vi "ActiveObjects_DynamicEvents.vi"(7 "Action":T2=enum."GeneratePattern", 8 "error in (no error)":errorcluster, 10 "DataIn":variant, 11 "ClassRefToActOn":refnum<vi>) -> (0 "error out":errorcluster, 1 "Name":string, 2 "DataOut":variant, 3 "Cancelled":bool)   [LabVIEW 2012]
uses:
  <resource>/Framework/Providers/Open_GDS/ClassProviders/Provider_BaseClassInterface/BaseProvider_SubVIs/BaseProvider_DesignPatternsActions.ctl
  <resource>/Framework/Providers/Open_GDS/ClassProviders/Common/LvClass_class/GDSLvClass_ProviderTypes.ctl
  <vilib>/picture/picture.llb/imagedata.ctl
  <resource>/Framework/Providers/Open_GDS/ClassProviders/Common/LvIcon_class/subvis/GDSLvIcon_TextDataType.ctl
  <resource>/Framework/Providers/Open_GDS/ClassProviders/Common/LvIcon_class/GDSLvIcon_WordCompressionType.ctl
  <resource>/Framework/Providers/Open_GDS/ClassProviders/Common/LvIcon_class/GDSLvIcon_TextAlignment.ctl
  <vilib>/Utility/lvfile.llb/NI_FileType.lvlib
panel:
  out "NameExist4":string
  in  "AddWindowControlVI":bool
  in  "WindowControlName":string caption="Enter process window control VI name"
  in  "ProcessCreation":T1(ring) caption="Process creation"
  out "NameExist1":string
  out "NameExist3":string
  out "NameExist2":string
  in  "AddInDestructor":bool
  in  "AddInConstructor":bool
  in  "StopName":string caption="Enter Stop Process Name"
  in  "StartName":string caption="Enter Start Process Name"
  in  "_Cancel":bool
  in  "_OK":bool
  in  "ProcessName":string caption="Enter Active Process Name"
  # "Active Object using Dymanic Events"
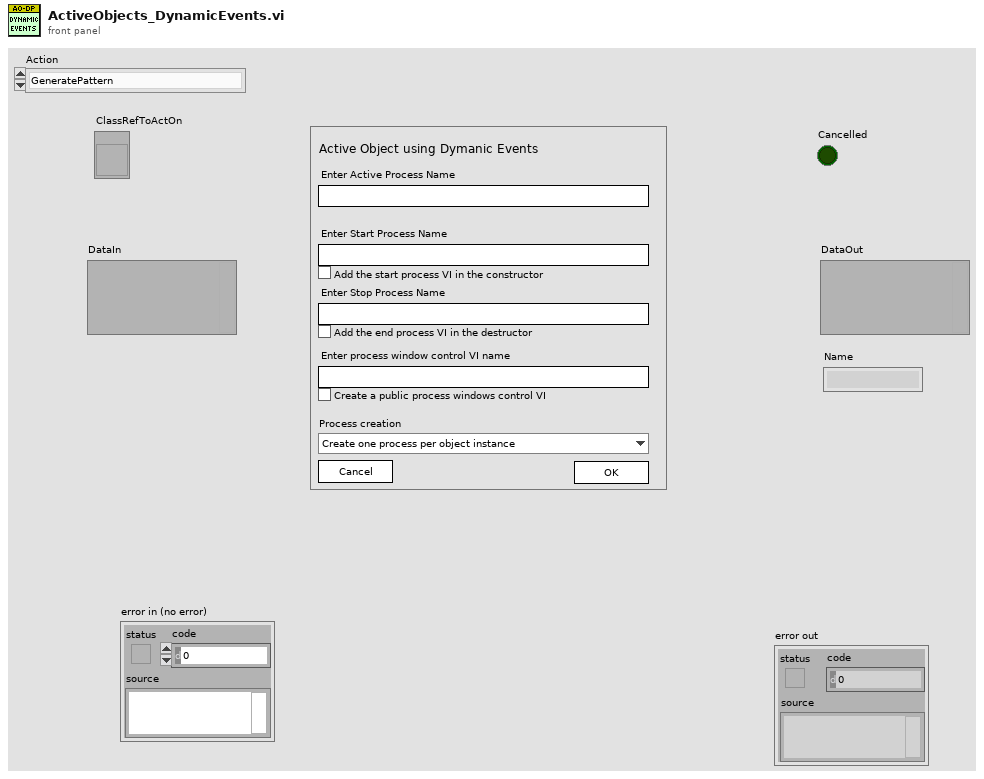
[diagram p1: front panel]
types:
  T1 = enum16{"Create one process per object instance", "Create only one process for this class"}
  T2 = typedef "BaseProvider_DesignPatternsActions.ctl" = enum16{"AddPatternDialog", "GeneratePattern", "RemovePattern", "CreatePatternMethod", "UpdatePattern"}
  T3 = typedef "GDSLvClass_ProviderTypes.ctl" = enum16{"UnKnown(LabVOOP)", "Native", "EndevoGOOP3", "OpenG(RootObject)", "OpenG(OpenG_Object)", "EndevoGOOP4", "JKI1"}
  T4 = cluster{"Data":cluster{"ProcessName":string, "StartName":string, "StopName":string, "AddInConstructor":bool, "AddInDestructor":bool, "ProcessCreation":enum16{"Create one process per object instance", "Create only one process for this class"}, "WindowControlName":string, "AddWindowControlVI":bool}, "ClassFolder":path, "SupportFolder":path, "ProcessCtl":refnum<vi>, "ProtectedFolder":refnum<vi>, "ProcessVI":refnum<vi>, "StartVI":refnum<vi>, "StopVI":refnum<vi>, "Application":refnum<vi>, "RepositoryVI":refnum<vi>, "ProcessIdRef":refnum<vi>, "ProcessRepository":path, "ClassProvider":T3, "TemplateName":string, "VI_ToFind":path, "MethodTemplate":path, "VI":refnum<vi>, "VI_ToFindSingleton":path, "Name":string, "WindowControlVI":refnum<vi>, "ClassType":enum16{"4x4x4", "6x8x6", "4x4x4_Singleton", "6x8x6_Singleton"}}
  T5 = cluster{"ProcessName":string, "StartName":string, "StopName":string, "AddInConstructor":bool, "AddInDestructor":bool, "ProcessCreation":enum16{"Create one process per object instance", "Create only one process for this class"}, "WindowControlName":string, "AddWindowControlVI":bool}
  T6 = cluster{"Cancelled":bool, "Files":path[], "ClassPath":path, "DataOut":variant, "Name":string}
  T7 = enum8{"Enabled", "Disabled", "Disabled and Grayed Out"}
  T8 = enum16{"4x4x4", "6x8x6", "4x4x4_Singleton", "6x8x6_Singleton"}
  T9 = enum32{"invalid VI type", "Standard VI", "Control VI", "Global VI", "Polymorphic VI", "Configuration VI", "SubSystem", "Facade VI", "Method VI"}
  T10 = typedef "GDSLvIcon_TextDataType.ctl" = cluster{"Text":string, "Allow Only Capital Chars":bool, "Compression":T11, "Alignment":T12}
  T11 = typedef "GDSLvIcon_WordCompressionType.ctl" = enum16{"Auto", "On", "Off"}
  T12 = typedef "GDSLvIcon_TextAlignment.ctl" = enum16{"Center", "Left", "Right"}
  T13 = typedef "imagedata.ctl" = cluster{"image type":i32, "image depth":i32, "image":u8[], "mask":u8[], "colors":u32[], "Rectangle":cluster{"left":i16, "top":i16, "right":i16, "bottom":i16}}
  T14 = typedef "GDSLvCLass_ClassSettingsType.ctl" = cluster{"ClassProviderName":string, "ClassTemplateUsed":string, "ClassTemplateVersion":string, "ClassDescription":string, "PlugIns":T15[], "ConnectorPanePattern":string}
  T15 = typedef "GDSLvClass_PlugIn.ctl" = cluster{"Type":T16, "ID":string, "Version":string, "Path":path, "Name":string, "Data":variant}
  T16 = typedef "GDSLvClass_PlugInTypes.ctl" = enum16{"DesignPattern", "MethodTypes"}
  T17 = enum32{"invalid scope", "public", "private", "protected"}[]
  T18 = enum16{"UINT8", "INT8", "UINT16", "INT16", "UINT32", "INT32", "UINT64", "INT64", "SGL", "DBL", "EXT", "CSG", "CDB", "CXT", "TimeStamp", "STRING", "PATH", "BOOL", "ENUM", "RefNum", "VIRefNum", "ClassRefNum", "Cluster", "Variant", "TypeRef", "Waveform", "LabVIEW Object", "Other"}[]
  T19 = typedef "GDSLvClass_IconSettingsType.ctl" = cluster{"Frame":u32, "Frame thickness":u8, "Header Background":u32, "Header Text":u32, "ColorPublic":u32, "ColorProtected":u32, "ColorPrivate":u32, "Body Text":u32, "ClassBodyIcon":string}
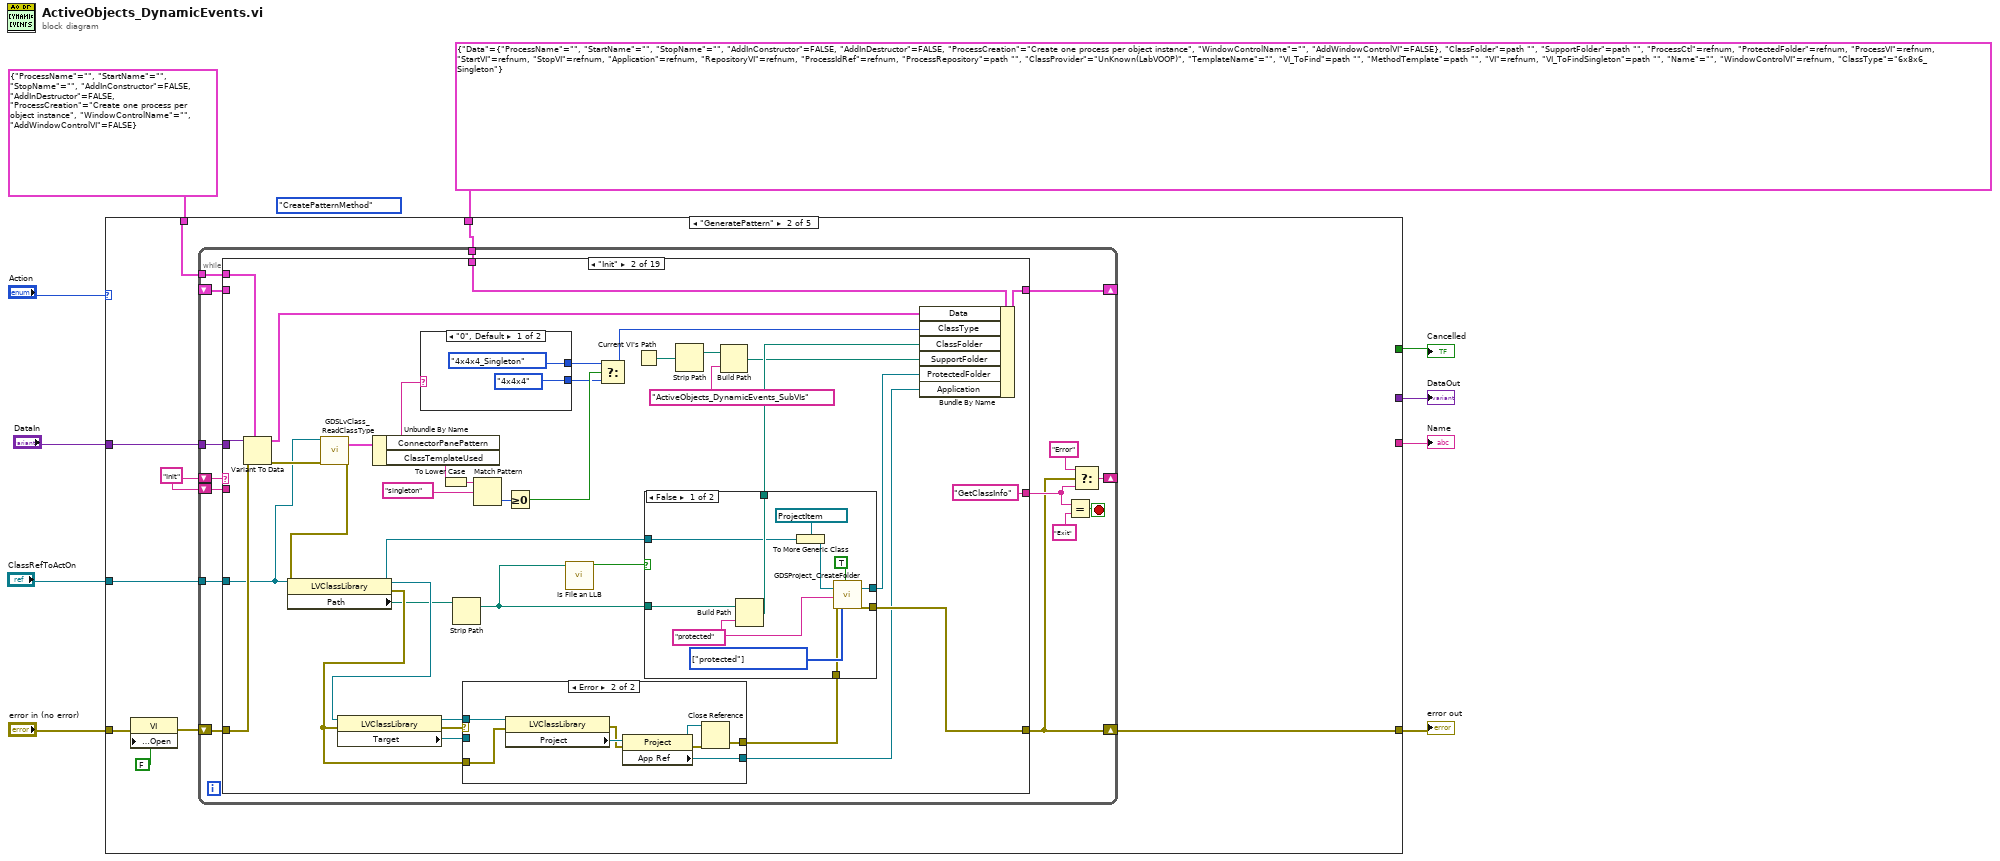
[diagram p0: block diagram]
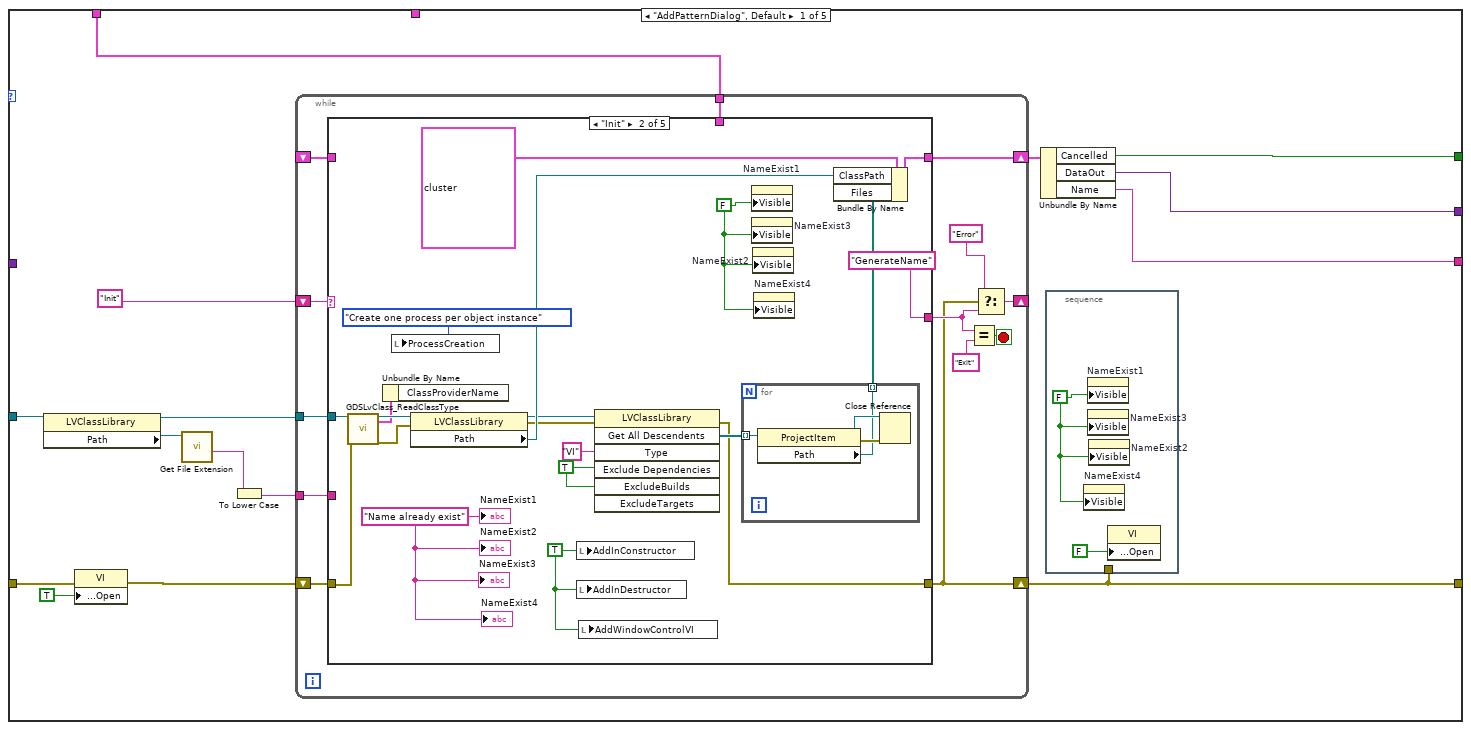
[diagram p2: hidden frame]
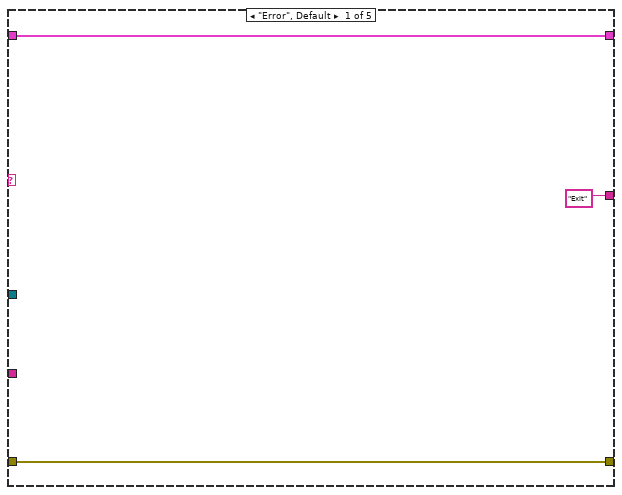
[diagram p3: hidden frame]
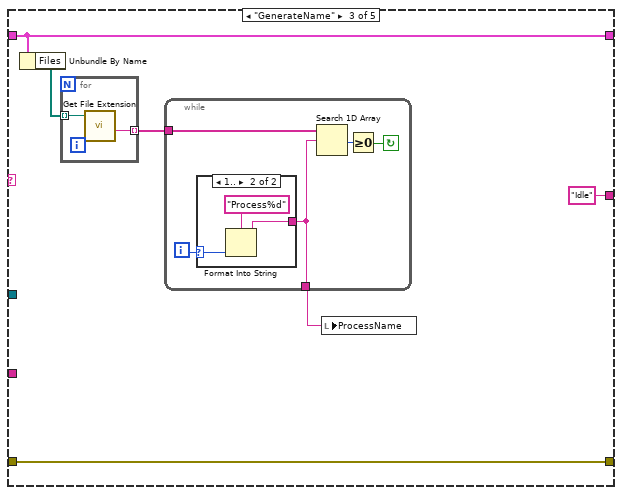
[diagram p4: hidden frame]
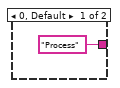
[diagram p5: hidden frame]
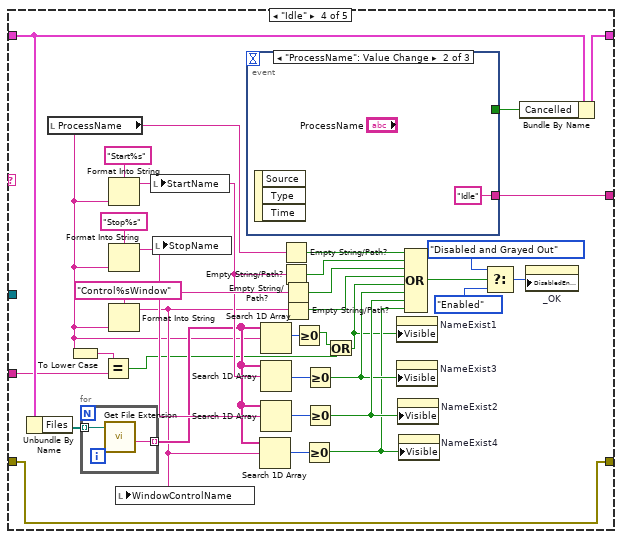
[diagram p6: hidden frame]
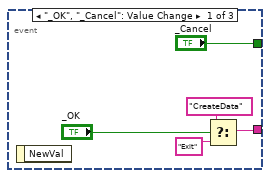
[diagram p7: hidden frame]
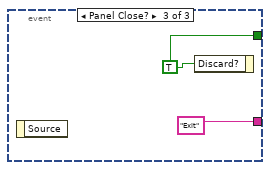
[diagram p8: hidden frame]
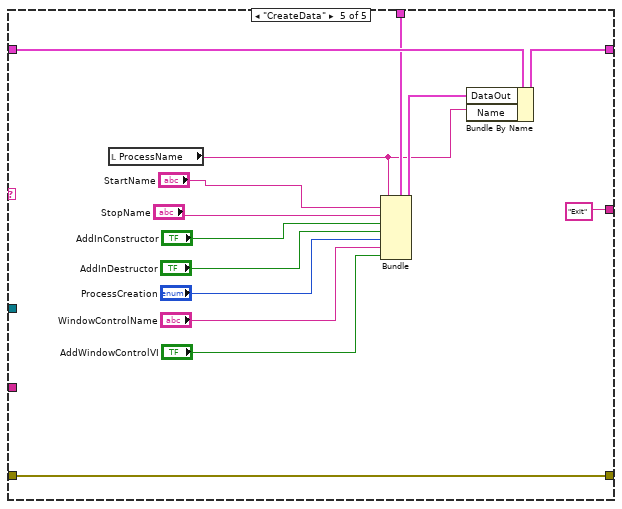
[diagram p9: hidden frame]
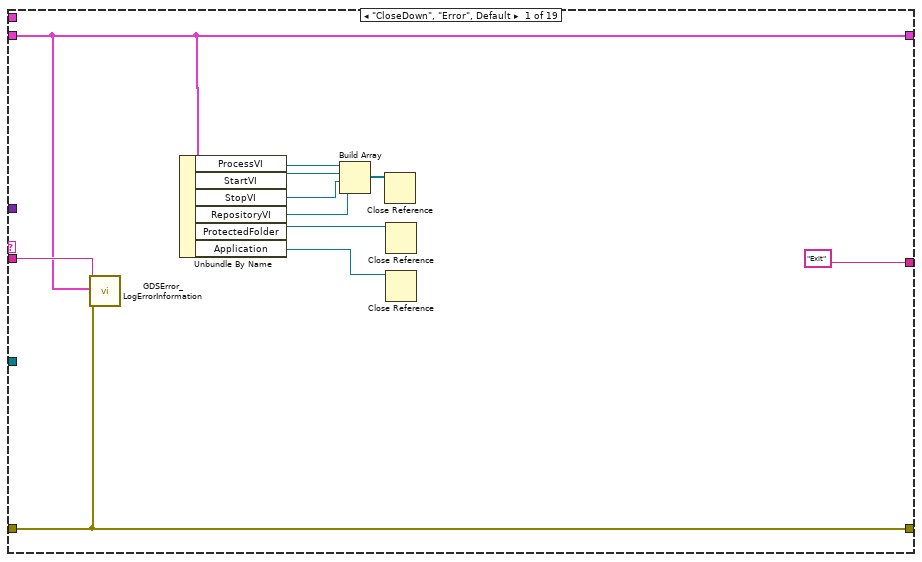
[diagram p10: hidden frame]
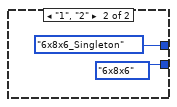
[diagram p11: hidden frame]
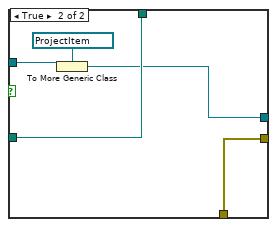
[diagram p12: hidden frame]
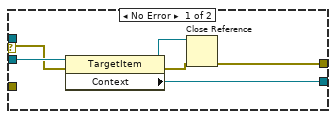
[diagram p13: hidden frame]
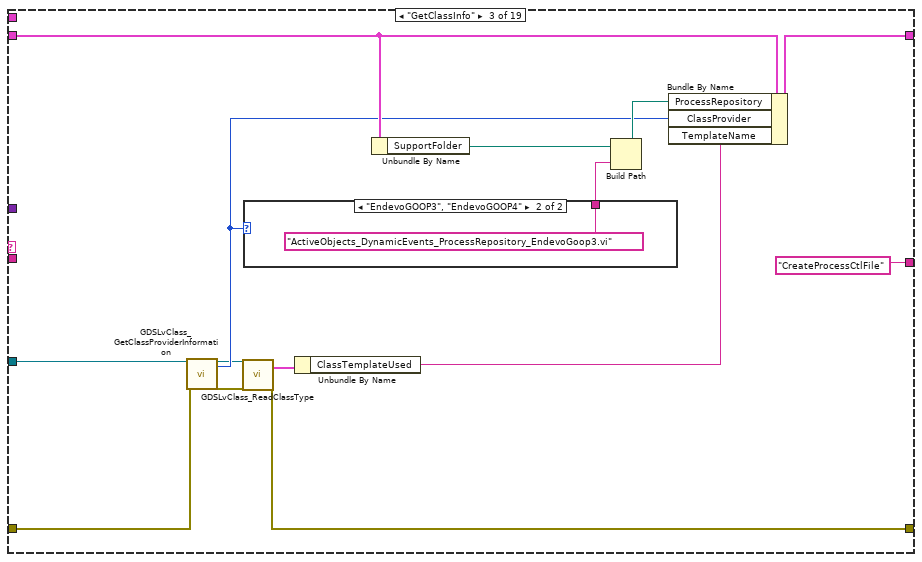
[diagram p14: hidden frame]
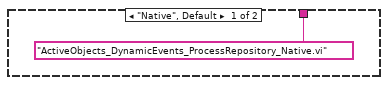
[diagram p15: hidden frame]
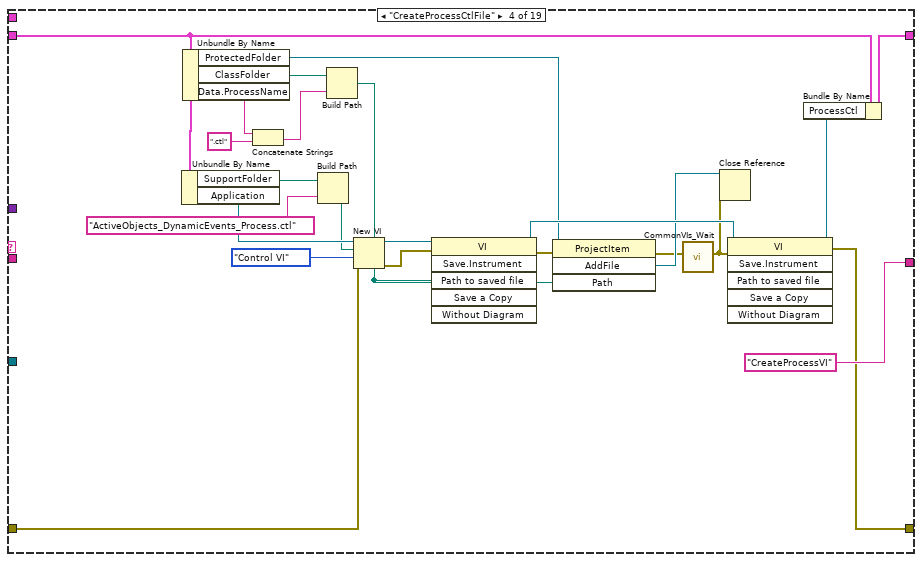
[diagram p16: hidden frame]
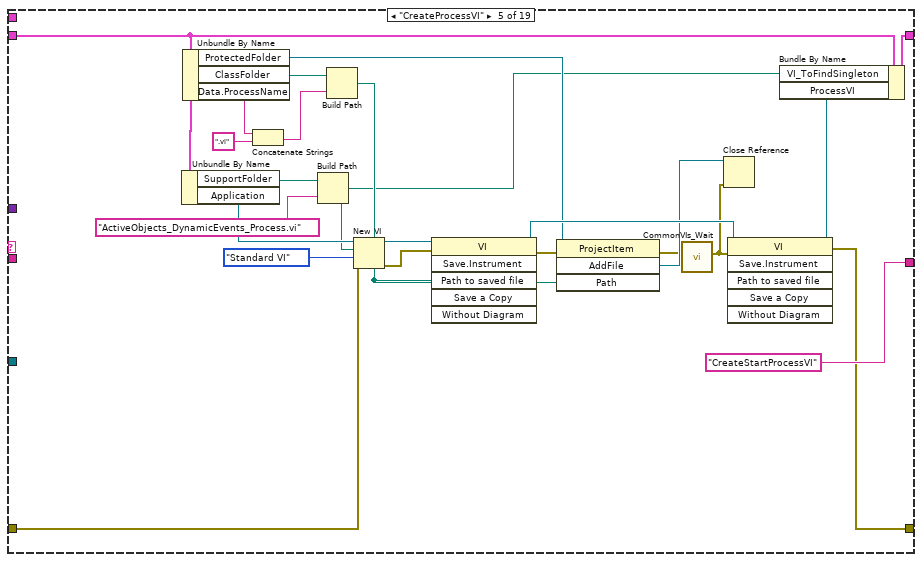
[diagram p17: hidden frame]
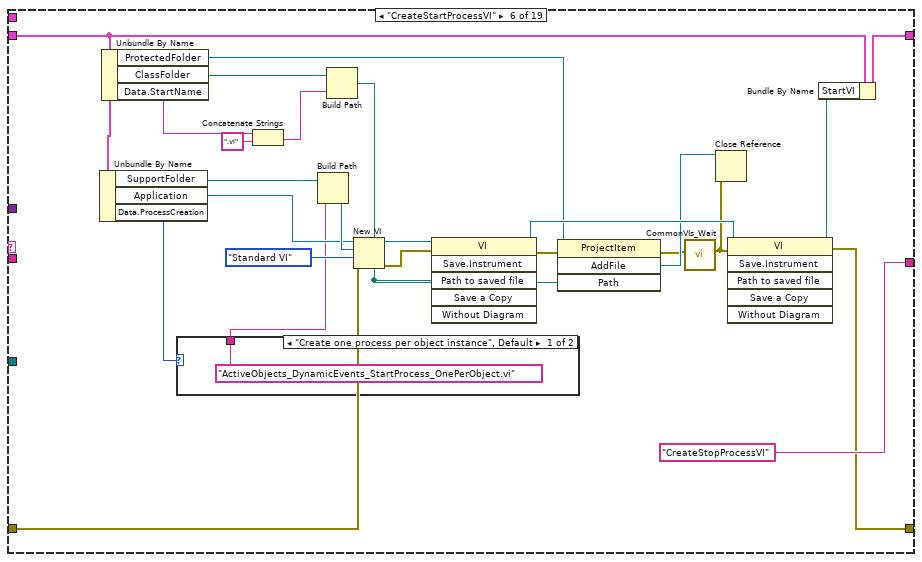
[diagram p18: hidden frame]
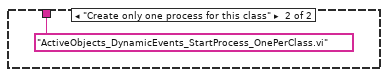
[diagram p19: hidden frame]
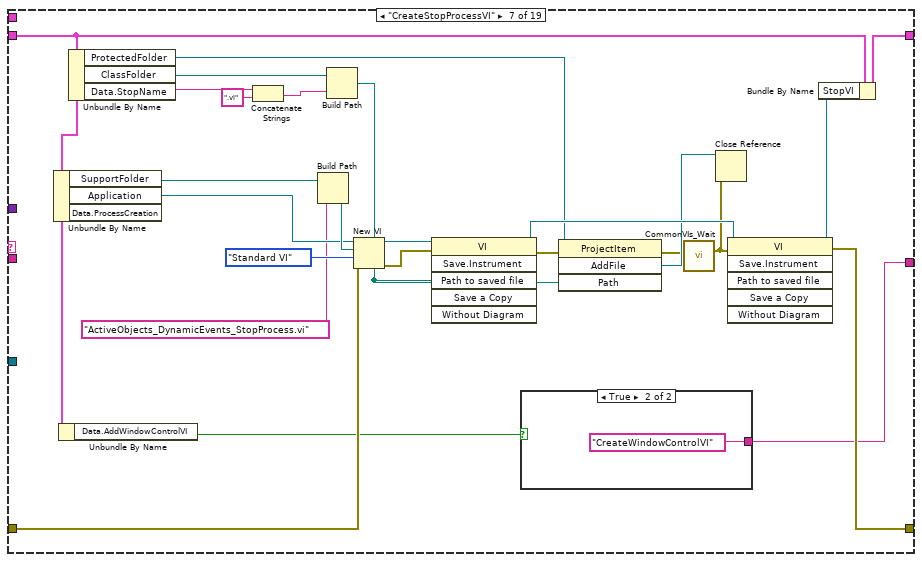
[diagram p20: hidden frame]
diagram:
  (unwired) BaseProvider_DesignPatternsActions."CreatePatternMethod" ("Action")
  n1 = case shown="\"GeneratePattern\"" "Action" {
    tunnel: "error in (no error)" -> [w24 w145 w768 w769 w775]
    tunnel: [w21 w151 w768 w769 w770] -> w8
    tunnel: "ClassRefToActOn" -> [w15 w147 _ _ w774]
    tunnel: [w19 _ _ _ _] -> w6
    tunnel: [w18 _ _ _ _] -> w5
    tunnel: T5 {"ProcessName"="", "StartName"="", "StopName"="", "AddInConstructor"=FALSE, "AddInDestructor"=FALSE, "ProcessCreation"=enum."Create one process per object instance", "WindowControlName"="", "AddWindowControlVI"=FALSE} ("output cluster") -> [w17 w149 _ _ w771]
    tunnel: "DataIn" -> [_ w150 _ _ w773]
    tunnel: T4 {"Data"={"ProcessName"="", "StartName"="", "StopName"="", "AddInConstructor"=FALSE, "AddInDestructor"=FALSE, "ProcessCreation"=enum."Create one process per object instance", "WindowControlName"="", "AddWindowControlVI"=FALSE}, "ClassFolder"=path "", "SupportFolder"=path "", "ProcessCtl"=refnum, "ProtectedFolder"=refnum, "ProcessVI"=refnum, "StartVI"=refnum, "StopVI"=refnum, "Application"=refnum, "RepositoryVI"=refnum, "ProcessIdRef"=refnum, "ProcessRepository"=path "", "ClassProvider"=enum."UnKnown(LabVOOP)", "TemplateName"="", "VI_ToFind"=path "", "MethodTemplate"=path "", "VI"=refnum, "VI_ToFindSingleton"=path "", "Name"="", "WindowControlVI"=refnum, "ClassType"=enum."6x8x6_Singleton"} -> [_ w148 _ _ w772]
    tunnel: [w16 _ _ _ _] -> w1
    frame "AddPatternDialog", Default {
      n2 = property class="LVClassLibrary"(reference=w15) -> (reference out=w14:refnum<vi>, "Path"=w13:path)  [unwired: 1 in, 1 out]
      n3 = property class="VI"(error in=w24, "Front Panel.Open"=TRUE ("Front Panel Window:Open")) -> (error out=w23:errorcluster)  [unwired: 1 in, 1 out]
      n4 = call <vilib>:"Get File Extension.vi"("file"=w13) -> ("filename without extension"=w11:string)  [unwired: 7 in, 3 out]
      n5 = To Lower Case(string=w11) -> (all lower case string=w12:string)
      n6 = while {
        shift-right: [w33] -> w21
        shift-left: w23 -> [w40]
        shift-right: [w38] -> _
        shift-left: "Init" -> [w39]
        shift-right: [w32] -> w20
        shift-left: _ -> [w31]
        tunnel: w14 -> [w30]
        tunnel: w17 -> [w29]
        tunnel: w12 -> [w28]
        stop <- w37 stop-if-true
        n7 = case shown="\"Init\"" w39 {
          tunnel: w40 -> [w43 w50 w68 w102 w136]
          tunnel: [w43 w59 w68 w102 w136] -> w33
          tunnel: ["Exit" "GenerateName" "Idle" w118 "Exit"] -> w34
          tunnel: [w41 w57 w69 w117 w138] -> w32
          tunnel: w31 -> [w41 _ w69 w112 w140]
          tunnel: w30 -> [_ w52 _ _ _]
          tunnel: w29 -> [_ _ _ _ w135]
          tunnel: w28 -> [_ _ _ w86 _]
          frame "Error", Default {
          }
          frame "Init" {
            w45 = "Name already exist" ("NameExist1")
            w44 = FALSE ("Visible")
            w46 = TRUE ("AddInConstructor")
            w61 = TRUE ("ExcludeDependencies")
            n8 = call <resource>:"GDSLvClass_ReadClassType.vi"("Class Refnum In"=w52, "error in (no error)"=w50) -> ("Class Refnum Out"=w51:refnum<vi>, "ClassSettings"=w48:T14, "error out"=w49:errorcluster)  [unwired: 15 in]
            n9 = Unbundle By Name(w48) -> ()  [unwired: 1 out]
            n10 = local write "ProcessCreation"(T1."Create one process per object instance" ("ProcessCreation")) -> ()
            n11 = property class="LVClassLibrary"(reference=w51, error in=w49) -> (reference out=w54:refnum<vi>, error out=w53:errorcluster, "Path"=w56:path)
            n12 = local write "AddInConstructor"(w46) -> ()
            n13 = local write "AddInDestructor"(w46) -> ()
            n14 = local write "AddWindowControlVI"(w46) -> ()
            n15 = invoke class="LVClassLibrary" method="Get All Descendents"(reference=w54, error in=w53, "Type"="VI", "Exclude Dependencies"=w61, "ExcludeBuilds"=w61) -> (error out=w59:errorcluster, "All Descendents"=w60:refnum<vi>[])  [unwired: 2 in, 5 out]
            n16 = for {
              tunnel: w60 -> [w67] mode=indexing
              tunnel: [w64] -> w55 mode=indexing
              n17 = property class="ProjectItem"(reference=w67) -> (reference out=w65:refnum<vi>, error out=w66:errorcluster, "Path"=w64:path)  [unwired: 1 in]
              n18 = Close Reference(reference=w65, error in (no error)=w66) -> ()  [unwired: 1 out]
            }
            n19 = property on="NameExist1" class="Str"("Visible"=w44) -> ()  [unwired: 2 in, 2 out]
            n20 = property on="NameExist3" class="Str"("Visible"=w44) -> ()  [unwired: 2 in, 2 out]
            n21 = property on="NameExist2" class="Str"("Visible"=w44) -> ()  [unwired: 2 in, 2 out]
            n22 = property on="NameExist4" class="Str"("Visible"=w44) -> ()  [unwired: 2 in, 2 out]
            n23 = Bundle By Name(cluster=T6 {"Cancelled"=FALSE, "Files"=[], "ClassPath"=path "", "DataOut"=variant, "Name"=""}, "ClassPath"=w56, "Files"=w55) -> (w57:T6)
            "NameExist2" <- w45
            "NameExist3" <- w45
            "NameExist1" <- w45
            "NameExist4" <- w45
          }
          frame "GenerateName" {
            n24 = Unbundle By Name(w69) -> ("Files"=w73:path[])
            n25 = for {
              tunnel: w73 -> [w84] mode=indexing
              tunnel: [w83] -> w72 mode=indexing
              n26 = call <vilib>:"Get File Extension.vi"("file"=w84) -> ("filename without extension"=w83:string)  [unwired: 7 in, 3 out]
            }
            n27 = while {
              tunnel: w72 -> [w77]
              tunnel: [w74] -> w71
              i -> [w78]
              stop <- w75 continue-if-true
              n28 = case shown="1.." w78 {
                selector: w78 -> [_ w81]
                tunnel: ["Process" ("format string") w80] -> w74
                frame 0, Default {
                }
                frame 1.. {
                  n29 = Format Into String(format string="Process%d", w81) -> (resulting string=w80:string)  [unwired: 2 in, 1 out]
                }
              }
              n30 = Search 1D Array(1D array=w77, element=w74) -> (index of element=w76:i32)  [unwired: 1 in]
              n31 = Greater Or Equal To 0?(x=w76) -> (x >= 0?=w75:bool)
            }
            n32 = local write "ProcessName"(w71) -> ()
          }
          frame "Idle" {
            n33 = Unbundle By Name(w112) -> ("Files"=w113:path[])
            n34 = local read "ProcessName"() -> (w88:string)
            n35 = To Lower Case(string=w88) -> (all lower case string=w87:string)
            n36 = for {
              tunnel: w113 -> [w120] mode=indexing
              tunnel: [w119] -> w99 mode=indexing
              n37 = call <vilib>:"Get File Extension.vi"("file"=w120) -> ("filename without extension"=w119:string)  [unwired: 7 in, 3 out]
            }
            n38 = Equal?(x=w87, y=w86) -> (x = y?=w85:bool)
            n39 = Format Into String(format string="Start%s", w88) -> (resulting string=w106:string)  [unwired: 2 in, 1 out]
            n40 = Format Into String(format string="Stop%s", w88) -> (resulting string=w107:string)  [unwired: 2 in, 1 out]
            n41 = Format Into String(format string="Control%sWindow", w88) -> (resulting string=w97:string)  [unwired: 2 in, 1 out]
            n42 = local write "WindowControlName"(w97) -> ()
            n43 = local write "StartName"(w106) -> ()
            n44 = local write "StopName"(w107) -> ()
            n45 = event shown="[1] \"ProcessName\": Value Change" {
              selector: _ -> [_ _ _]
              dyn-events: _ -> [_ _ _]
              timeout: _ -> [_ _ _]
              tunnel: [w124 "Idle" "Exit"] -> w118
              tunnel: ["_Cancel" _ w127] -> w116
              event "_OK", "_Cancel": Value Change {
                n46 = event-data() -> ()  [unwired: 1 in, 1 out]
                n47 = Select(t="CreateData", s="_OK", f="Exit") -> (s? t:f=w124:string)
              }
              event "ProcessName": Value Change {
                n48 = event-data() -> ()  [unwired: 1 in, 3 out]
              }
              event Panel Close? {
                w127 = TRUE ("Discard?")
                n49 = event-data() -> ()  [unwired: 1 in, 1 out]
                n50 = event-data("Discard?"=w127) -> ()  [unwired: 1 in, 1 out]
              }
            }
            n51 = Search 1D Array(1D array=w99, element=w97) -> (index of element=w100:i32)  [unwired: 1 in]
            n52 = Search 1D Array(1D array=w99, element=w88) -> (index of element=w111:i32)  [unwired: 1 in]
            n53 = Search 1D Array(1D array=w99, element=w106) -> (index of element=w110:i32)  [unwired: 1 in]
            n54 = Search 1D Array(1D array=w99, element=w107) -> (index of element=w109:i32)  [unwired: 1 in]
            n55 = Empty String/Path?(string/path=w88) -> (empty?=w103:bool)
            n56 = Empty String/Path?(string/path=w106) -> (empty?=w104:bool)
            n57 = Empty String/Path?(string/path=w107) -> (empty?=w105:bool)
            n58 = Empty String/Path?(string/path=w97) -> (empty?=w96:bool)
            n59 = Greater Or Equal To 0?(x=w111) -> (x >= 0?=w90:bool)
            n60 = Greater Or Equal To 0?(x=w100) -> (x >= 0?=w95:bool)
            n61 = Greater Or Equal To 0?(x=w110) -> (x >= 0?=w101:bool)
            n62 = Greater Or Equal To 0?(x=w109) -> (x >= 0?=w108:bool)
            n63 = Or(x=w90, y=w85) -> (x .or. y?=w89:bool)
            n64 = property on="NameExist1" class="Str"("Visible"=w89) -> ()  [unwired: 2 in, 2 out]
            n65 = property on="NameExist3" class="Str"("Visible"=w101) -> ()  [unwired: 2 in, 2 out]
            n66 = property on="NameExist2" class="Str"("Visible"=w108) -> ()  [unwired: 2 in, 2 out]
            n67 = property on="NameExist4" class="Str"("Visible"=w95) -> ()  [unwired: 2 in, 2 out]
            n68 = Compound Arithmetic op=OR(w103, w104, w105, w96, w89, w101, w108, w95) -> (w94:bool)
            n69 = Select(t=T7."Disabled and Grayed Out" ("Disabled"), s=w94, f=T7."Enabled" ("Disabled")) -> (s? t:f=w93:T7)
            n70 = Bundle By Name(cluster=w112, "Cancelled"=w116) -> (w117:T6)
            n71 = property on="_OK" class="Bool"("DisabledEnum"=w93) -> ()  [unwired: 2 in, 2 out]
          }
          frame "CreateData" {
            n72 = local read "ProcessName"() -> (w133:string)
            n73 = Bundle(cluster=w135, "ProcessName"=w133, "StartName"="StartName", "StopName"="StopName", "AddInConstructor"="AddInConstructor", "AddInDestructor"="AddInDestructor", "ProcessCreation"="ProcessCreation", "WindowControlName"="WindowControlName", "AddWindowControlVI"="AddWindowControlVI") -> (w139:T5)
            n74 = Bundle By Name(cluster=w140, "DataOut"=w139, "Name"=w133) -> (w138:T6)
          }
        }
        n75 = Equal?(x=w34, y="Exit") -> (x = y?=w37:bool)
        n76 = Select(t="Error", s=w33, f=w34) -> (s? t:f=w38:string)
      }
      n77 = Unbundle By Name(w20) -> ("Cancelled"=w19:bool, "DataOut"=w18:variant, "Name"=w16:string)
      n78 = stacked-sequence {
        tunnel: w21 -> [_]
        frame #0 {
          w26 = FALSE ("Visible")
          n79 = property on="NameExist4" class="Str"("Visible"=w26) -> ()  [unwired: 2 in, 2 out]
          n80 = property on="NameExist1" class="Str"("Visible"=w26) -> ()  [unwired: 2 in, 2 out]
          n81 = property on="NameExist3" class="Str"("Visible"=w26) -> ()  [unwired: 2 in, 2 out]
          n82 = property on="NameExist2" class="Str"("Visible"=w26) -> ()  [unwired: 2 in, 2 out]
          n83 = property class="VI"("Front Panel.Open"=FALSE ("Front Panel Window:Open")) -> ()  [unwired: 2 in, 2 out]
        }
      }
    }
    frame "GeneratePattern" {
      w143 = "Init"
      n84 = property class="VI"(error in=w145, "Front Panel.Open"=FALSE ("Front Panel Window:Open")) -> (error out=w144:errorcluster)  [unwired: 1 in, 1 out]
      n85 = while {
        shift-right: [w159] -> w151
        shift-left: w144 -> [w166]
        shift-right: [w164] -> _
        shift-left: w143 -> [w165]
        shift-right: [w158] -> _
        shift-left: _ -> [w157]
        tunnel: w150 -> [w156]
        tunnel: w149 -> [w155]
        tunnel: w148 -> [w154]
        tunnel: w147 -> [w153]
        shift-left: w143 -> [w152]
        stop <- w163 stop-if-true
        n86 = case shown="\"Init\"" w165 {
          tunnel: w166 -> [w169 w208 w260 w284 w308 w333 w360 w389 w419 w435 w446 w486 w512 w545 w554 w580 w650 w703 w765]
          tunnel: [w169 w202 w251 w271 w295 w321 w349 w376 w410 w424 w443 w468 w500 w536 w553 w579 w648 w701 w764] -> w159
          tunnel: ["Exit" "GetClassInfo" "CreateProcessCtlFile" "CreateProcessVI" "CreateStartProcessVI" "CreateStopProcessVI" w342 "CreateProcessRepositoryVI" w403 "UpdateOORefInVIs" w442 "UpdateVIs" "UpdateRepositoryStaticVI" w547 "UpdateIcons" "UpdateCreate?" "UpdateDestroy?" "SaveAll" "CloseDown"] -> w160
          tunnel: [w172 w213 w254 w274 w298 w324 w351 w378 w412 w428 w450 w484 w492 w530 w550 w582 w646 w699 w767] -> w158
          tunnel: w157 -> [w172 _ w257 w275 w299 w315 w344 w379 w401 w429 w450 w484 w492 w530 w550 w582 w646 w699 w767]
          tunnel: w156 -> [_ w212 _ _ _ _ _ _ _ _ _ _ _ _ _ _ _ _ _]
          tunnel: w155 -> [_ w211 _ _ _ _ _ _ _ _ _ _ _ _ _ _ _ _ _]
          tunnel: w154 -> [_ w210 _ _ _ _ _ _ _ _ _ _ _ _ _ _ _ _ _]
          tunnel: w153 -> [_ w188 w261 _ _ _ _ w370 _ w426 w445 w474 _ _ w551 w586 w645 w698 w763]
          tunnel: w152 -> [w176 _ _ _ _ _ _ _ _ _ _ _ _ _ _ _ _ _ _]
          frame "CloseDown", "Error", Default {
            n87 = call <resource>:"GDSError_LogErrorInformation.vi"("State"=w176, "LocalVariableData"=w172, "error in (no error)"=w169) -> ()  [unwired: 16 in, 1 out]
            n88 = Unbundle By Name(w172) -> ("ProcessVI"=w175:refnum<vi>, "StartVI"=w174:refnum<vi>, "StopVI"=w173:refnum<vi>, "RepositoryVI"=w171:refnum<vi>, "ProtectedFolder"=w168:refnum<vi>, "Application"=w167:refnum<vi>)
            n89 = Build Array(w175, w174, w173, w171) -> (w170:refnum<vi>[])
            n90 = Close Reference(reference=w170) -> ()  [unwired: 1 in, 1 out]
            n91 = Close Reference(reference=w168) -> ()  [unwired: 1 in, 1 out]
            n92 = Close Reference(reference=w167) -> ()  [unwired: 1 in, 1 out]
          }
          frame "Init" {
            n93 = Variant To Data(error in=w208, type=w211, Variant=w212) -> (data=w209:T5, error out=w190:errorcluster)
            n94 = call <resource>:"GDSLvClass_ReadClassType.vi"("Class Refnum In"=w188, "error in (no error)"=w190) -> ("ClassSettings"=w182:T14, "error out"=w189:errorcluster)  [unwired: 15 in, 1 out]
            n95 = property class="LVClassLibrary"(reference=w188, error in=w189) -> (reference out=w196:refnum<vi>, error out=w197:errorcluster, "Path"=w193:path)
            n96 = property class="LVClassLibrary"(reference=w196, error in=w197) -> (reference out=w200:refnum<vi>, error out=w198:errorcluster, "Target"=w199:refnum<vi>)
            n97 = Unbundle By Name(w182) -> ("ConnectorPanePattern"=w187:string, "ClassTemplateUsed"=w186:string)
            n98 = case shown="\"0\", Default" w187 {
              tunnel: [T8."4x4x4" ("ClassType") T8."6x8x6" ("ClassType")] -> w180
              tunnel: [T8."4x4x4_Singleton" ("ClassType") T8."6x8x6_Singleton" ("ClassType")] -> w179
              frame "0", Default {
              }
              frame "1", "2" {
              }
            }
            n99 = To Lower Case(string=w186) -> (all lower case string=w184:string)
            n100 = Strip Path(path=w193) -> (stripped path=w191:path)  [unwired: 1 out]
            n101 = case shown="Error" w198 {
              selector: w198 -> [w236 _]
              tunnel: w199 -> [w240 _]
              tunnel: [w239 w242] -> w195
              tunnel: [w235 w243] -> w194
              tunnel: w200 -> [_ w248]
              tunnel: w197 -> [_ w247]
              frame No Error {
                n102 = property class="TargetItem"(reference=w240, error in=w236) -> (reference out=w237:refnum<vi>, error out=w238:errorcluster, "Context"=w239:refnum<vi>)
                n103 = Close Reference(reference=w237, error in (no error)=w238) -> (error out=w235:errorcluster)
              }
              frame Error {
                n104 = property class="LVClassLibrary"(reference=w248, error in=w247) -> (error out=w241:errorcluster, "Project"=w246:refnum<vi>)  [unwired: 1 out]
                n105 = property class="Project"(reference=w246, error in=w241) -> (reference out=w244:refnum<vi>, error out=w245:errorcluster, "App Ref"=w242:refnum<vi>)
                n106 = Close Reference(reference=w244, error in (no error)=w245) -> (error out=w243:errorcluster)
              }
            }
            n107 = Match Pattern(string=w184, regular expression="singleton" ("search string")) -> (offset past match=w185:i32)  [unwired: 1 in, 3 out]
            n108 = Greater Or Equal To 0?(x=w185) -> (x >= 0?=w181:bool)
            n109 = call <vilib>:"Is File an LLB.vi"("path"=w191) -> ("Is LLB?"=w192:bool)  [unwired: 9 in, 1 out]
            n110 = Select(t=w179, s=w181, f=w180) -> (s? t:f=w178:T8)
            n111 = Current VI's Path() -> (path=w206:path)
            n112 = case shown="False" w192 {
              tunnel: [w224 w231] -> w207
              tunnel: [w223 w232] -> w202
              tunnel: [w222 w230] -> w201
              tunnel: w196 -> [w221 w233]
              tunnel: w194 -> [w220 w232]
              tunnel: w191 -> [w219 w231]
              frame False {
                w227 = T17 [enum."protected"] items=["invalid scope", "public", "private", "protected"] ("FolderScope")
                w226 = "protected" ("name or relative path")
                n113 = Build Path(base path=w219, name or relative path=w226) -> (appended path=w224:path)
                n114 = To More Generic Class(target class=refnum<vi> refnum ("AddItem"), reference=w221) -> (generic class reference=w228:refnum<vi>)
                n115 = call <resource>:"GDSProject_CreateFolder.vi"("Project Item To Create Folder Below(Use MyComputer if not wired)"=w228, "FolderName"=w226, "error in (no error)"=w220, "FolderScope"=w227, "CreateThePhysicalFolderIfPossible(False)"=TRUE) -> ("ItemOut"=w222:refnum<vi>, "error out"=w223:errorcluster)  [unwired: 11 in, 2 out]
              }
              frame True {
                n116 = To More Generic Class(target class=refnum<vi> refnum ("AddItem"), reference=w233) -> (generic class reference=w230:refnum<vi>)
              }
            }
            n117 = Strip Path(path=w206) -> (stripped path=w205:path)  [unwired: 1 out]
            n118 = Build Path(base path=w205, name or relative path="ActiveObjects_DynamicEvents_SubVIs") -> (appended path=w203:path)
            n119 = Bundle By Name(cluster=w210, "Data"=w209, "ClassType"=w178, "ClassFolder"=w207, "SupportFolder"=w203, "ProtectedFolder"=w201, "Application"=w195) -> (w213:T4)
          }
          frame "GetClassInfo" {
            n120 = call <resource>:"GDSLvClass_GetClassProviderInformation.vi"("Class Refnum In"=w261, "error in (no error)"=w260) -> ("Class Refnum Out"=w253:refnum<vi>, "ClassProvider"=w255:T3, "error out"=w252:errorcluster)  [unwired: 15 in]
            n121 = call <resource>:"GDSLvClass_ReadClassType.vi"("Class Refnum In"=w253, "error in (no error)"=w252) -> ("ClassSettings"=w250:T14, "error out"=w251:errorcluster)  [unwired: 15 in, 1 out]
            n122 = case shown="\"EndevoGOOP3\", \"EndevoGOOP4\"" w255 {
              tunnel: ["ActiveObjects_DynamicEvents_ProcessRepository_Native.vi" ("name or relative path") "ActiveObjects_DynamicEvents_ProcessRepository_EndevoGoop3.vi" ("name or relative path")] -> w258
              frame "Native", Default {
              }
              frame "EndevoGOOP3", "EndevoGOOP4" {
              }
            }
            n123 = Unbundle By Name(w250) -> ("ClassTemplateUsed"=w249:string)
            n124 = Unbundle By Name(w257) -> ("SupportFolder"=w259:path)
            n125 = Build Path(base path=w259, name or relative path=w258) -> (appended path=w256:path)
            n126 = Bundle By Name(cluster=w257, "ProcessRepository"=w256, "ClassProvider"=w255, "TemplateName"=w249) -> (w254:T4)
          }
          frame "CreateProcessCtlFile" {
            n127 = Unbundle By Name(w275) -> ("SupportFolder"=w280:path, "Application"=w269:refnum<vi>)
            n128 = Unbundle By Name(w275) -> ("ProtectedFolder"=w270:refnum<vi>, "ClassFolder"=w288:path, "Data.ProcessName"=w287:string)
            n129 = Concatenate Strings(w287, ".ctl" ("string")) -> (w285:string)
            n130 = Build Path(base path=w280, name or relative path="ActiveObjects_DynamicEvents_Process.ctl") -> (appended path=w267:path)
            n131 = Build Path(base path=w288, name or relative path=w285) -> (appended path=w277:path)
            n132 = New VI(8:w284, 9:T9."Control VI" ("vi type (standard vi)"), 10:w267, 11:w269) -> (0:w281:errorcluster, 3:w282:refnum<vi>)  [unwired: 3 in]
            n133 = invoke class="VI" method="Save.Instrument"(reference=w282, error in=w281, "Path to saved file"=w277) -> (reference out=w276:refnum<vi>, error out=w278:errorcluster)  [unwired: 3 in, 4 out]
            n134 = invoke class="ProjectItem" method="AddFile"(reference=w270, error in=w278, "Path"=w277) -> (error out=w266:errorcluster, "AddFile"=w268:refnum<vi>)  [unwired: 1 in, 2 out]
            n135 = call <resource>:"CommonVIs_Wait.vi"("error in"=w266) -> ("error out"=w265:errorcluster)  [unwired: 9 in]
            n136 = Close Reference(reference=w268, error in (no error)=w265) -> ()  [unwired: 1 out]
            n137 = invoke class="VI" method="Save.Instrument"(reference=w276, error in=w265) -> (reference out=w273:refnum<vi>, error out=w271:errorcluster)  [unwired: 4 in, 4 out]
            n138 = Bundle By Name(cluster=w275, "ProcessCtl"=w273) -> (w274:T4)
          }
          frame "CreateProcessVI" {
            n139 = Unbundle By Name(w299) -> ("SupportFolder"=w304:path, "Application"=w293:refnum<vi>)
            n140 = Unbundle By Name(w299) -> ("ProtectedFolder"=w294:refnum<vi>, "ClassFolder"=w312:path, "Data.ProcessName"=w311:string)
            n141 = Concatenate Strings(w311, ".vi" ("string")) -> (w309:string)
            n142 = Build Path(base path=w304, name or relative path="ActiveObjects_DynamicEvents_Process.vi") -> (appended path=w291:path)
            n143 = Build Path(base path=w312, name or relative path=w309) -> (appended path=w301:path)
            n144 = New VI(8:w308, 9:T9."Standard VI" ("vi type (standard vi)"), 10:w291, 11:w293) -> (0:w305:errorcluster, 3:w306:refnum<vi>)  [unwired: 3 in]
            n145 = invoke class="VI" method="Save.Instrument"(reference=w306, error in=w305, "Path to saved file"=w301) -> (reference out=w300:refnum<vi>, error out=w302:errorcluster)  [unwired: 3 in, 4 out]
            n146 = invoke class="ProjectItem" method="AddFile"(reference=w294, error in=w302, "Path"=w301) -> (error out=w290:errorcluster, "AddFile"=w292:refnum<vi>)  [unwired: 1 in, 2 out]
            n147 = call <resource>:"CommonVIs_Wait.vi"("error in"=w290) -> ("error out"=w289:errorcluster)  [unwired: 9 in]
            n148 = Close Reference(reference=w292, error in (no error)=w289) -> ()  [unwired: 1 out]
            n149 = invoke class="VI" method="Save.Instrument"(reference=w300, error in=w289) -> (reference out=w297:refnum<vi>, error out=w295:errorcluster)  [unwired: 4 in, 4 out]
            n150 = Bundle By Name(cluster=w299, "VI_ToFindSingleton"=w291, "ProcessVI"=w297) -> (w298:T4)
          }
          frame "CreateStartProcessVI" {
            n151 = Unbundle By Name(w315) -> ("SupportFolder"=w329:path, "Application"=w319:refnum<vi>, "Data.ProcessCreation"=w318:T1)
            n152 = Unbundle By Name(w315) -> ("ProtectedFolder"=w320:refnum<vi>, "ClassFolder"=w337:path, "Data.StartName"=w336:string)
            n153 = case shown="\"Create one process per object instance\", Default" w318 {
              tunnel: ["ActiveObjects_DynamicEvents_StartProcess_OnePerObject.vi" ("name or relative path") "ActiveObjects_DynamicEvents_StartProcess_OnePerClass.vi" ("name or relative path")] -> w317
              frame "Create one process per object instance", Default {
              }
              frame "Create only one process for this class" {
              }
            }
            n154 = Concatenate Strings(w336, ".vi" ("string")) -> (w334:string)
            n155 = Build Path(base path=w329, name or relative path=w317) -> (appended path=w328:path)
            n156 = Build Path(base path=w337, name or relative path=w334) -> (appended path=w326:path)
            n157 = New VI(8:w333, 9:T9."Standard VI" ("vi type (standard vi)"), 10:w328, 11:w319) -> (0:w330:errorcluster, 3:w331:refnum<vi>)  [unwired: 3 in]
            n158 = invoke class="VI" method="Save.Instrument"(reference=w331, error in=w330, "Path to saved file"=w326) -> (reference out=w325:refnum<vi>, error out=w327:errorcluster)  [unwired: 3 in, 4 out]
            n159 = invoke class="ProjectItem" method="AddFile"(reference=w320, error in=w327, "Path"=w326) -> (error out=w314:errorcluster, "AddFile"=w316:refnum<vi>)  [unwired: 1 in, 2 out]
            n160 = call <resource>:"CommonVIs_Wait.vi"("error in"=w314) -> ("error out"=w313:errorcluster)  [unwired: 9 in]
            n161 = Close Reference(reference=w316, error in (no error)=w313) -> ()  [unwired: 1 out]
            n162 = invoke class="VI" method="Save.Instrument"(reference=w325, error in=w313) -> (reference out=w323:refnum<vi>, error out=w321:errorcluster)  [unwired: 4 in, 4 out]
            n163 = Bundle By Name(cluster=w315, "StartVI"=w323) -> (w324:T4)
          }
          frame "CreateStopProcessVI" {
            n164 = Unbundle By Name(w344) -> ("SupportFolder"=w356:path, "Application"=w347:refnum<vi>)  [unwired: 1 out]
            n165 = Unbundle By Name(w344) -> ("Data.AddWindowControlVI"=w343:bool)
            n166 = Unbundle By Name(w344) -> ("ProtectedFolder"=w348:refnum<vi>, "ClassFolder"=w364:path, "Data.StopName"=w363:string)
            n167 = Concatenate Strings(w363, ".vi" ("string")) -> (w361:string)
            n168 = Build Path(base path=w356, name or relative path="ActiveObjects_DynamicEvents_StopProcess.vi") -> (appended path=w355:path)
            n169 = Build Path(base path=w364, name or relative path=w361) -> (appended path=w353:path)
            n170 = New VI(8:w360, 9:T9."Standard VI" ("vi type (standard vi)"), 10:w355, 11:w347) -> (0:w357:errorcluster, 3:w358:refnum<vi>)  [unwired: 3 in]
            n171 = invoke class="VI" method="Save.Instrument"(reference=w358, error in=w357, "Path to saved file"=w353) -> (reference out=w352:refnum<vi>, error out=w354:errorcluster)  [unwired: 3 in, 4 out]
            n172 = case shown="True" w343 {
              tunnel: ["CreateProcessRepositoryVI" "CreateWindowControlVI"] -> w342
              frame False {
              }
              frame True {
              }
            }
            n173 = invoke class="ProjectItem" method="AddFile"(reference=w348, error in=w354, "Path"=w353) -> (error out=w341:errorcluster, "AddFile"=w346:refnum<vi>)  [unwired: 1 in, 2 out]
            n174 = call <resource>:"CommonVIs_Wait.vi"("error in"=w341) -> ("error out"=w340:errorcluster)  [unwired: 9 in]
            n175 = Close Reference(reference=w346, error in (no error)=w340) -> ()  [unwired: 1 out]
            n176 = invoke class="VI" method="Save.Instrument"(reference=w352, error in=w340) -> (reference out=w350:refnum<vi>, error out=w349:errorcluster)  [unwired: 4 in, 4 out]
            n177 = Bundle By Name(cluster=w344, "StopVI"=w350) -> (w351:T4)
          }
          frame "CreateWindowControlVI" {
            n178 = Unbundle By Name(w379) -> ("ClassFolder"=w393:path, "Data.WindowControlName"=w392:string)  [unwired: 1 out]
            n179 = Unbundle By Name(w379) -> ("SupportFolder"=w385:path, "Application"=w375:refnum<vi>, "ClassType"=w372:T8)
            n180 = To More Generic Class(target class=refnum<vi> refnum ("AddItem"), reference=w370) -> (generic class reference=w369:refnum<vi>)
            n181 = case shown="\"4x4x4_Singleton\"" w372 {
              tunnel: ["ActiveObjects_DynamicEvents_ControlWindow_4x4x4.vi" ("name or relative path") "ActiveObjects_DynamicEvents_ControlWindow_6x8x6.vi" ("name or relative path") "ActiveObjects_DynamicEvents_ControlWindow_4x4x4_Singleton.vi" ("name or relative path") "ActiveObjects_DynamicEvents_ControlWindow_6x8x6_Singleton.vi" ("name or relative path")] -> w384
              frame "4x4x4", Default {
              }
              frame "6x8x6" {
              }
              frame "4x4x4_Singleton" {
              }
              frame "6x8x6_Singleton" {
              }
            }
            n182 = Concatenate Strings(w392, ".vi" ("string")) -> (w390:string)
            n183 = Build Path(base path=w385, name or relative path=w384) -> (appended path=w383:path)
            n184 = Build Path(base path=w393, name or relative path=w390) -> (appended path=w381:path)
            n185 = New VI(8:w389, 9:T9."Standard VI" ("vi type (standard vi)"), 10:w383, 11:w375) -> (0:w386:errorcluster, 3:w387:refnum<vi>)  [unwired: 3 in]
            n186 = invoke class="VI" method="Save.Instrument"(reference=w387, error in=w386, "Path to saved file"=w381) -> (reference out=w380:refnum<vi>, error out=w382:errorcluster)  [unwired: 3 in, 4 out]
            n187 = invoke class="ProjectItem" method="AddFile"(reference=w369, error in=w382, "Path"=w381) -> (error out=w368:errorcluster, "AddFile"=w374:refnum<vi>)  [unwired: 1 in, 2 out]
            n188 = call <resource>:"CommonVIs_Wait.vi"("error in"=w368) -> ("error out"=w367:errorcluster)  [unwired: 9 in]
            n189 = Close Reference(reference=w374, error in (no error)=w367) -> ()  [unwired: 1 out]
            n190 = invoke class="VI" method="Save.Instrument"(reference=w380, error in=w367) -> (reference out=w377:refnum<vi>, error out=w376:errorcluster)  [unwired: 4 in, 4 out]
            n191 = Bundle By Name(cluster=w379, "WindowControlVI"=w377) -> (w378:T4)
          }
          frame "CreateProcessRepositoryVI" {
            n192 = Unbundle By Name(w401) -> ("ClassProvider"=w400:T3)
            n193 = Unbundle By Name(w401) -> ("ProcessRepository"=w402:path, "Application"=w408:refnum<vi>)
            n194 = Unbundle By Name(w401) -> ("ProtectedFolder"=w409:refnum<vi>, "ClassFolder"=w420:path, "Data.ProcessName"=w407:string)
            n195 = Format Into String(format string="%sRepository.vi", w407) -> (resulting string=w405:string)  [unwired: 2 in, 1 out]
            n196 = New VI(8:w419, 9:T9."Standard VI" ("vi type (standard vi)"), 10:w402, 11:w408) -> (0:w416:errorcluster, 3:w417:refnum<vi>)  [unwired: 3 in]
            n197 = Build Path(base path=w420, name or relative path=w405) -> (appended path=w414:path)
            n198 = invoke class="VI" method="Save.Instrument"(reference=w417, error in=w416, "Path to saved file"=w414) -> (reference out=w413:refnum<vi>, error out=w415:errorcluster)  [unwired: 3 in, 4 out]
            n199 = invoke class="ProjectItem" method="AddFile"(reference=w409, error in=w415, "Path"=w414) -> (error out=w399:errorcluster, "AddFile"=w404:refnum<vi>)  [unwired: 1 in, 2 out]
            n200 = case shown="Default" w400 {
              tunnel: ["UpdateOORefInVIs" "AddCtlToAttribute"] -> w403
              frame Default {
              }
              frame "UnKnown(LabVOOP)", "Native" {
              }
            }
            n201 = call <resource>:"CommonVIs_Wait.vi"("error in"=w399) -> ("error out"=w398:errorcluster)  [unwired: 9 in]
            n202 = Close Reference(reference=w404, error in (no error)=w398) -> ()  [unwired: 1 out]
            n203 = invoke class="VI" method="Save.Instrument"(reference=w413, error in=w398) -> (reference out=w411:refnum<vi>, error out=w410:errorcluster)  [unwired: 4 in, 4 out]
            n204 = Bundle By Name(cluster=w401, "RepositoryVI"=w411) -> (w412:T4)
          }
          frame "AddCtlToAttribute" {
            w433 = T18 [enum."UINT32"] items=["UINT8", "INT8", "UINT16", "INT16", "UINT32", "INT32", "UINT64", "INT64", "SGL", "DBL", "EXT", "CSG", "CDB", "CXT", "TimeStamp", "STRING", "PATH", "BOOL", "ENUM", "RefNum", "VIRefNum", "ClassRefNum", "Cluster", "Variant", "TypeRef", "Waveform", "LabVIEW Object", "Other"] ("DataTypes")
            n205 = call <resource>:"Scripting_PlaceControlsInClassAttribute.vi"("ClassRefnum"=w426, "DeleteAllCurrentAttributesFirst(True)"=FALSE, "ControlNames"=string[] ["ProcessId:Process#No"], "DataTypes"=w433, "error in"=w435, "DeleteReferencesToCreatedAttributes(True)"=FALSE) -> ("ControlsCreated"=w430:refnum<vi>[], "error out"=w425:errorcluster)  [unwired: 7 in, 1 out]
            n206 = Index Array(array=w430) -> (element=w427:refnum<vi>)  [unwired: 1 in]
            n207 = call <resource>:"GDSLvClass_SaveEverythingInClass.vi"("ClassRefIn"=w426, "error in"=w425) -> ("error out"=w424:errorcluster)  [unwired: 16 in, 1 out]
            n208 = Bundle By Name(cluster=w429, "ProcessIdRef"=w427) -> (w428:T4)
          }
          frame "UpdateOORefInVIs" {
            n209 = Unbundle By Name(w450) -> ("Data.AddWindowControlVI"=w436:bool, "ProcessVI"=w449:refnum<vi>, "StartVI"=w448:refnum<vi>, "StopVI"=w447:refnum<vi>, "RepositoryVI"=w439:refnum<vi>, "WindowControlVI"=w437:refnum<vi>, "ClassProvider"=w438:T3)
            n210 = property class="LVClassLibrary"(reference=w445) -> ("Path"=w441:path)  [unwired: 1 in, 2 out]
            n211 = case shown="False" w436 {
              tunnel: w449 -> [w456 w461]
              tunnel: w448 -> [w455 w460]
              tunnel: w447 -> [w454 w459]
              tunnel: [w453 w458] -> w444
              tunnel: w439 -> [w452 w457]
              tunnel: w437 -> [w451 _]
              frame True {
                n212 = Build Array(w456, w455, w454, w452, w451) -> (w453:refnum<vi>[])
              }
              frame False {
                n213 = Build Array(w461, w460, w459, w457) -> (w458:refnum<vi>[])
              }
            }
            n214 = Path To String(path=w441) -> (string=w440:string)
            n215 = for {
              tunnel: w444 -> [w464] mode=indexing
              shift-right: [w467] -> w443
              shift-left: w446 -> [w466]
              tunnel: w440 -> [w465]
              n216 = call <resource>:"Scripting_ReplaceOORef.vi"("ViRef"=w464, "NewLvClassFile(ProjectPath or LvClassPath)"=w465, "error in (no error)"=w466) -> ("error out"=w467:errorcluster)  [unwired: 16 in]
            }
            n217 = case shown="Default" w438 {
              tunnel: ["UpdateVIs" "RenameProcessIdControl"] -> w442
              frame Default {
              }
              frame "UnKnown(LabVOOP)", "Native" {
              }
            }
          }
          frame "RenameProcessIdControl" {
            w479 = T18 [enum."UINT32"] items=["UINT8", "INT8", "UINT16", "INT16", "UINT32", "INT32", "UINT64", "INT64", "SGL", "DBL", "EXT", "CSG", "CDB", "CXT", "TimeStamp", "STRING", "PATH", "BOOL", "ENUM", "RefNum", "VIRefNum", "ClassRefNum", "Cluster", "Variant", "TypeRef", "Waveform", "LabVIEW Object", "Other"] ("DataTypes")
            n218 = Unbundle By Name(w484) -> ("ProcessIdRef"=w487:refnum<vi>, "Data.ProcessName"=w482:string)
            n219 = Format Into String(format string="ProcessId:%s", w482) -> (resulting string=w481:string)  [unwired: 2 in, 1 out]
            n220 = property class="Ctl"(reference=w487, error in=w486, "Label.Text"=w481) -> (error out=w476:errorcluster)  [unwired: 1 out]
            n221 = call <resource>:"Scripting_PlaceControlsInClassAttribute.vi"("ClassRefnum"=w474, "DeleteAllCurrentAttributesFirst(True)"=FALSE, "ControlNames"=string[] ["DummyStringThatShouldBeDeleted"], "DataTypes"=w479, "error in"=w476, "DeleteReferencesToCreatedAttributes(True)"=FALSE) -> ("ControlsCreated"=w473:refnum<vi>[], "error out"=w475:errorcluster)  [unwired: 7 in, 1 out]
            n222 = Index Array(array=w473) -> (element=w472:refnum<vi>)  [unwired: 1 in]
            n223 = call <resource>:"GDSLvClass_SaveEverythingInClass.vi"("ClassRefIn"=w474, "ForceResaving(False)"=TRUE, "error in"=w475) -> ("ClassRefOut"=w470:refnum<vi>, "error out"=w469:errorcluster)  [unwired: 15 in]
            n224 = invoke class="Ctl" method="Delete"(reference=w472, error in=w469) -> (error out=w471:errorcluster)  [unwired: 1 in, 2 out]
            n225 = call <resource>:"GDSLvClass_SaveEverythingInClass.vi"("ClassRefIn"=w470, "error in"=w471) -> ("error out"=w468:errorcluster)  [unwired: 16 in, 1 out]
          }
          frame "UpdateVIs" {
            n226 = Unbundle By Name(w492) -> ("Data.AddWindowControlVI"=w489:bool, "ProcessVI"=w504:refnum<vi>, "StartVI"=w503:refnum<vi>, "StopVI"=w502:refnum<vi>, "WindowControlVI"=w490:refnum<vi>, "RepositoryVI"=w498:refnum<vi>)
            n227 = Unbundle By Name(w492) -> ("SupportFolder"=w494:path)
            n228 = Unbundle By Name(w492) -> ("RepositoryVI"=w513:refnum<vi>, "ProcessCtl"=w507:refnum<vi>)
            n229 = Unbundle By Name(w492) -> ("SupportFolder"=w511:path)
            n230 = case shown="False" w489 {
              tunnel: w504 -> [w519 w523]
              tunnel: w503 -> [w518 w522]
              tunnel: w502 -> [w517 w521]
              tunnel: [w516 w520] -> w499
              tunnel: w490 -> [w515 _]
              frame True {
                n231 = Build Array(w519, w518, w517, w515) -> (w516:refnum<vi>[])
              }
              frame False {
                n232 = Build Array(w523, w522, w521) -> (w520:refnum<vi>[])
              }
            }
            n233 = Build Path(base path=w494, name or relative path="ActiveObjects_DynamicEvents_ProcessRepository_Native.vi") -> (appended path=w491:path)
            n234 = property class="VI"(reference=w507) -> ("Path"=w506:path)  [unwired: 1 in, 2 out]
            n235 = property class="VI"(reference=w498) -> ("Path"=w497:path)  [unwired: 1 in, 2 out]
            n236 = Build Path(base path=w511, name or relative path="ActiveObjects_DynamicEvents_Process.ctl") -> (appended path=w509:path)
            n237 = Build Array(w509) -> (w508:path[])
            n238 = Build Array(w506) -> (w505:path[])
            n239 = Build Array(w497) -> (w496:path[])
            n240 = Build Array(w491) -> (w495:path[])
            n241 = call <resource>:"Scripting_ReplaceVisAndControls.vi"("ViRef"=w513, "OldVIsAndControls"=w508, "NewVIsAndControls"=w505, "error in (no error)"=w512) -> ("error out"=w501:errorcluster)  [unwired: 14 in, 1 out]
            n242 = for {
              shift-right: [w527] -> w500
              shift-left: w501 -> [w528]
              tunnel: w499 -> [w526] mode=indexing
              tunnel: w496 -> [w525]
              tunnel: w495 -> [w524]
              n243 = call <resource>:"Scripting_ReplaceVisAndControls.vi"("ViRef"=w526, "OldVIsAndControls"=w524, "NewVIsAndControls"=w525, "error in (no error)"=w528) -> ("error out"=w527:errorcluster)  [unwired: 14 in, 1 out]
            }
          }
          frame "UpdateRepositoryStaticVI" {
            w542 = refnum<vi> refnum  # StaticVIReference
            n244 = Unbundle By Name(w530) -> ("RepositoryVI"=w546:refnum<vi>)
            n245 = Unbundle By Name(w530) -> ("ClassType"=w529:T8)
            n246 = Unbundle By Name(w530) -> ("ClassFolder"=w535:path, "Data.ProcessName"=w534:string)
            n247 = Concatenate Strings(w534, ".vi" ("string")) -> (w532:string)
            n248 = Build Path(base path=w535, name or relative path=w532) -> (appended path=w531:path)
            n249 = call <resource>:"Scripting_FindNodeOnDiagram.vi"("ViRef(Ignored If Not Wired)"=w546, "NodeTypesToSearchFor"=string[] ["StaticVIReference"], "error in (no error)"=w545) -> ("Nodes"=w538:refnum<vi>[], "error out"=w537:errorcluster)  [unwired: 15 in]
            n250 = Index Array(array=w538) -> (element=w543:refnum<vi>)  [unwired: 1 in]
            n251 = To More Specific Class(target class=w542, reference=w543, error in=w537) -> (specific class reference=w541:refnum<vi>, error out=w540:errorcluster)
            n252 = property class="StatVIRef"(reference=w541, error in=w540, "Path"=w531) -> (error out=w539:errorcluster)  [unwired: 1 out]
            n253 = case shown="\"4x4x4_Singleton\", \"6x8x6_Singleton\"" w529 {
              tunnel: ["UpdateIcons" "FixSingletonCodeWithGetInstance"] -> w547
              frame Default {
              }
              frame "4x4x4_Singleton", "6x8x6_Singleton" {
              }
            }
            n254 = Close Reference(reference=w538, error in (no error)=w539) -> (error out=w536:errorcluster)
          }
          frame "FixSingletonCodeWithGetInstance" {
            n255 = Unbundle By Name(w550) -> ("VI_ToFindSingleton"=w559:path, "WindowControlVI"=w555:refnum<vi>)
            n256 = Build Array(w559) -> (w558:path[])
            n257 = call <resource>:"GDSLvClass_GetClassMethod.vi"("Class Refnum In"=w551, "VINames"=string[] ["GetInstance.vi$"] ("VIsToSerachFor/ViName"), "error in (no error)"=w554) -> ("ViPaths"=w565:path[], "error out"=w560:errorcluster)  [unwired: 13 in, 2 out]
            n258 = call <resource>:"Scripting_FindVisOnDiagram.vi"("ViRef"=w555, "VIsToSerachFor/ViName"=w558, "error in (no error)"=w560) -> ("VisFound"=w562:refnum<vi>[], "error out"=w561:errorcluster)  [unwired: 15 in]
            n259 = Index Array(array=w565) -> (element=w557:path)  [unwired: 1 in]
            n260 = Index Array(array=w562) -> (element=w563:refnum<vi>)  [unwired: 1 in]
            n261 = invoke class="GObj" method="Replace"(reference=w563, error in=w561, "Path"=w557) -> (error out=w556:errorcluster, "Replace"=w564:refnum<vi>)  [unwired: 3 in, 4 out]
            n262 = Close Reference(reference=w562, error in (no error)=w556) -> ()  [unwired: 1 out]
            n263 = Close Reference(reference=w564, error in (no error)=w556) -> (error out=w553:errorcluster)
          }
          frame "UpdateIcons" {
            w603 = u8 32 ("x")
            n264 = Unbundle By Name(w582) -> ("Data.AddWindowControlVI"=w568:bool, "ProcessVI"=w585:refnum<vi>, "StartVI"=w584:refnum<vi>, "StopVI"=w583:refnum<vi>, "RepositoryVI"=w574:refnum<vi>, "WindowControlVI"=w570:refnum<vi>, "Data.ProcessName"=w573:string, "Data.StartName"=w577:string, "Data.StopName"=w576:string, "Data.WindowControlName"=w569:string)
            n265 = property class="LVClassLibrary"(reference=w586, error in=w580) -> (reference out=w591:refnum<vi>, error out=w587:errorcluster, "Member Data"=w589:refnum<vi>)
            n266 = call <resource>:"GDSLvIcon_AnalyseViIcon.vi"("ViRef/LvCLassRef/LvLibRef/ViPath"=w589, "error in (no error)"=w587) -> ("HeaderIcon"=w592:u8[][], "error out"=w588:errorcluster)  [unwired: 6 in, 10 out]
            n267 = case shown="True" w568 {
              tunnel: w585 -> [w613 w618]
              tunnel: w584 -> [w612 w617]
              tunnel: w583 -> [w611 w616]
              tunnel: [w610 w615] -> w578
              tunnel: w574 -> [w609 w614]
              tunnel: w570 -> [w608 _]
              frame True {
                n268 = Build Array(w613, w612, w611, w609, w608) -> (w610:refnum<vi>[])
              }
              frame False {
                n269 = Build Array(w618, w617, w616, w614) -> (w615:refnum<vi>[])
              }
            }
            n270 = Close Reference(reference=w589, error in (no error)=w588) -> (error out=w590:errorcluster)
            n271 = Format Into String(format string="%sRepository", w573) -> (resulting string=w572:string)  [unwired: 2 in, 1 out]
            n272 = Array Size(array=w592) -> (size(s)=w598:i32[])
            n273 = call <resource>:"GDSLvClass_ReadClassColors.vi"("Library Refnum"=w591, "error in (no error)"=w590) -> ("LvClassIconSettings"=w594:T19, "error out"=w581:errorcluster)  [unwired: 12 in, 4 out]
            n274 = Unbundle By Name(w594) -> ("Frame"=w597:u32, "Body Text"=w596:u32, "Frame thickness"=w593:u8)
            n275 = Build Array(w573, w577, w576, w572, w569) -> (w575:string[])
            n276 = Unbundle By Name(w594) -> ("ColorPublic"=w567:u32, "ColorProtected"=w595:u32)
            n277 = Index Array(array=w598) -> (element #1=w600:i32)  [unwired: 2 in, 1 out]
            n278 = Multiply(x=w593, y=u8 2) -> (x*y=w601:u8)
            n279 = Add(x=w600, y=w601) -> (x+y=w602:i32)
            n280 = Increment(x=w602) -> (x+1=w604:i32)
            n281 = Subtract(x=w603, y=w604) -> (x-y=w605:i32)
            n282 = Subtract(x=w603, y=w601) -> (x-y=w606:u8)
            n283 = for {
              tunnel: w606 -> [w644]
              tunnel: w605 -> [w643]
              tunnel: w597 -> [w640]
              tunnel: w596 -> [w639]
              tunnel: w595 -> [w620]
              tunnel: w593 -> [w638]
              tunnel: w592 -> [w637]
              shift-right: [w627] -> w579
              shift-left: w581 -> [w629]
              tunnel: w578 -> [w626] mode=indexing
              tunnel: w575 -> [w625] mode=indexing
              tunnel: w567 -> [w621]
              i -> [w624]
              n284 = Bundle By Name(cluster=T10 {"Text"="", "Allow Only Capital Chars"=TRUE, "Compression"=enum."Auto", "Alignment"=enum."Center"} ("Text"), "Text"=w625) -> (w642:T10)
              n285 = Equal?(x=w624, y=4) -> (x = y?=w622:bool)
              n286 = Select(t=w621, s=w622, f=w620) -> (s? t:f=w619:u32)
              n287 = call <resource>:"GDSLvIcon_GenerateIconText.vi"("Text"=w642, "TextPixelHeight(5-30)"=w643, "Foreground color"=w639, "Background color"=w619, "error in (no error)"=w629, "Text Pixel width(32-FrameThicknes*2))"=w644) -> ("TextOut"=w636:u8[][], "error out"=w628:errorcluster)  [unwired: 9 in, 3 out]
              n288 = call <resource>:"GDSLvIcon_CreateIconPicture.vi"("FrameColor"=w640, "FrameThickness(1)"=w638, "HeaderIconIn"=w637, "BodyIconIn"=w636, "error in (no error)"=w628) -> ("WholeIconOut"=w631:u8[][], "error out"=w634:errorcluster)  [unwired: 9 in, 4 out]
              n289 = Reshape Array(w631, 1024 ("dimension size")) -> (w633:u8[])
              n290 = Bundle By Name(cluster=T13 {"image type"=0, "image depth"=8, "image"=[], "mask"=[], "colors"=[], "Rectangle"={"left"=0, "top"=0, "right"=32, "bottom"=32}} ("image data"), "image"=w633) -> (w635:T13)
              n291 = invoke class="VI" method="VI Icon.Set from Image Data"(reference=w626, error in=w634, "ImageData"=w635) -> (error out=w627:errorcluster)  [unwired: 3 in, 5 out]
            }
          }
          frame "UpdateCreate?" {
            n292 = Unbundle By Name(w646) -> ("Data.AddInConstructor"=w649:bool)
            n293 = case shown="True" w649 {
              tunnel: w650 -> [w651 w672]
              tunnel: [w651 w671] -> w648
              tunnel: w646 -> [_ w670]
              tunnel: w645 -> [_ w666]
              frame False {
              }
              frame True {
                n294 = Unbundle By Name(w670) -> ("Application"=w659:refnum<vi>, "StartVI"=w669:refnum<vi>, "ClassProvider"=w667:T3, "TemplateName"=w656:string)
                n295 = property class="LVClassLibrary"(reference=w666) -> ("Path"=w665:path)  [unwired: 1 in, 2 out]
                n296 = To Lower Case(string=w656) -> (all lower case string=w655:string)
                n297 = Strip Path(path=w665) -> (stripped path=w664:path)  [unwired: 1 out]
                n298 = Match Pattern(string=w655, regular expression="singleton") -> (offset past match=w653:i32)  [unwired: 1 in, 3 out]
                n299 = Greater Or Equal To 0?(x=w653) -> (x >= 0?=w652:bool)
                n300 = property class="VI"(reference=w669) -> ("Path"=w668:path)  [unwired: 1 in, 2 out]
                n301 = case shown="\"EndevoGOOP3\", \"EndevoGOOP4\"" w667 {
                  tunnel: ["*Init.vi" w693 "*_Create.vi" "Constructor*.vi"] -> w663
                  tunnel: w652 -> [_ w692 _ _]
                  frame "Native", Default {
                  }
                  frame "EndevoGOOP3", "EndevoGOOP4" {
                    n302 = case shown="True" w692 {
                      tunnel: ["*Init.vi" "*_Create.vi"] -> w693
                      frame True {
                      }
                      frame False {
                      }
                    }
                  }
                  frame "OpenG(RootObject)" {
                  }
                  frame "OpenG(OpenG_Object)" {
                  }
                }
                n303 = call <vilib>:"Recursive File List.vi"("pattern"=w663, "Treat LLBs as Folders?"=TRUE, "Folder Path"=w664) -> ("All Files in Dir"=w661:path[])  [unwired: 4 in, 4 out]
                n304 = Index Array(array=w661) -> (element=w658:path)  [unwired: 1 in]
                n305 = call <vilib>:"Check if File or Folder Exists.vi"("path"=w658) -> ("file or folder exists?"=w660:bool)  [unwired: 8 in, 2 out]
                n306 = case shown="True" w660 {
                  tunnel: w672 -> [w673 w674]
                  tunnel: [w673 w675] -> w671
                  tunnel: w668 -> [_ w686]
                  tunnel: w659 -> [_ w684]
                  tunnel: w658 -> [_ w683]
                  tunnel: "The \"Start Process VI\" could not automatically be placed in the Create/Construct method.\nPlease add this method manually." ("message") -> [_ w677]
                  frame False {
                  }
                  frame True {
                    n307 = Open VI Reference(application reference (local)=w684, vi path=w683, error in (no error)=w674) -> (vi reference=w682:refnum<vi>, error out=w685:errorcluster)  [unwired: 3 in]
                    n308 = call <resource>:"Scripting_AddVIInsideNoErrorCase.vi"("ViToModify"=w682, "VIToAdd"=w686, "error in (no error)"=w685, "AddVIOnLeftSideCaseStructure"=FALSE, "OnlyReference"=FALSE) -> ("error out"=w681:errorcluster)  [unwired: 14 in]
                    n309 = invoke class="VI" method="Save.Instrument"(reference=w682, error in=w681) -> (reference out=w679:refnum<vi>, error out=w680:errorcluster)  [unwired: 4 in, 4 out]
                    n310 = Close Reference(reference=w679, error in (no error)=w680) -> (error out=w676:errorcluster)
                    n311 = case shown="Error" w676 {
                      selector: w676 -> [w688 _]
                      tunnel: [w688 w690] -> w675
                      tunnel: w674 -> [_ w690]
                      tunnel: w677 -> [_ w689]
                      frame No Error {
                      }
                      frame Error {
                        n312 = One Button Dialog(message=w689) -> ()  [unwired: 1 in, 1 out]
                      }
                    }
                  }
                }
              }
            }
          }
          frame "UpdateDestroy?" {
            n313 = Unbundle By Name(w699) -> ("Data.AddInDestructor"=w702:bool)
            n314 = case shown="True" w702 {
              tunnel: w703 -> [w704 w714]
              tunnel: [w704 w713] -> w701
              tunnel: w699 -> [_ w712]
              tunnel: w698 -> [_ w711]
              frame False {
              }
              frame True {
                n315 = Unbundle By Name(w712) -> ("Application"=w716:refnum<vi>, "StopVI"=w725:refnum<vi>, "ClassProvider"=w723:T3, "TemplateName"=w706:string)
                n316 = To Lower Case(string=w706) -> (all lower case string=w709:string)
                n317 = property class="LVClassLibrary"(reference=w711) -> ("Path"=w722:path)  [unwired: 1 in, 2 out]
                n318 = Strip Path(path=w722) -> (stripped path=w721:path)  [unwired: 1 out]
                n319 = Match Pattern(string=w709, regular expression="singleton") -> (offset past match=w707:i32)  [unwired: 1 in, 3 out]
                n320 = Greater Or Equal To 0?(x=w707) -> (x >= 0?=w705:bool)
                n321 = case shown="\"EndevoGOOP3\", \"EndevoGOOP4\"" w723 {
                  tunnel: ["CleanUp.vi" w757 "Destroy.vi" "Destructor*.vi"] -> w720
                  tunnel: w705 -> [_ w756 _ _]
                  frame "Native", Default {
                  }
                  frame "EndevoGOOP3", "EndevoGOOP4" {
                    n322 = case shown="False" w756 {
                      tunnel: ["*CleanUp.vi" "Destroy.vi"] -> w757
                      frame True {
                      }
                      frame False {
                      }
                    }
                  }
                  frame "OpenG(RootObject)" {
                  }
                  frame "OpenG(OpenG_Object)" {
                  }
                }
                n323 = call <vilib>:"Recursive File List.vi"("pattern"=w720, "Treat LLBs as Folders?"=TRUE, "Folder Path"=w721) -> ("All Files in Dir"=w718:path[])  [unwired: 4 in, 4 out]
                n324 = property class="VI"(reference=w725) -> ("Path"=w724:path)  [unwired: 1 in, 2 out]
                n325 = Index Array(array=w718) -> (element=w715:path)  [unwired: 1 in]
                n326 = call <vilib>:"Check if File or Folder Exists.vi"("path"=w715) -> ("file or folder exists?"=w717:bool)  [unwired: 8 in, 2 out]
                n327 = case shown="True" w717 {
                  tunnel: w714 -> [w726 w729]
                  tunnel: [w726 w730] -> w713
                  tunnel: w724 -> [_ w739]
                  tunnel: w716 -> [_ w737]
                  tunnel: w715 -> [_ w736]
                  tunnel: "The \"Stop Process VI\" could not automatically be placed in the Destroy/Destruct method.\nPlease add this method manually before the object is destroyed." ("message") -> [_ w728]
                  tunnel: w705 -> [_ w727]
                  frame False {
                  }
                  frame True {
                    n328 = Open VI Reference(application reference (local)=w737, vi path=w736, error in (no error)=w729) -> (vi reference=w735:refnum<vi>, error out=w738:errorcluster)  [unwired: 3 in]
                    n329 = case shown="True" w727 {
                      tunnel: w739 -> [w744 w751]
                      tunnel: w738 -> [w743 w750]
                      tunnel: w735 -> [w742 w748]
                      tunnel: [w741 w749] -> w734
                      frame False {
                        n330 = call <resource>:"Scripting_AddVIInsideNoErrorCase.vi"("ViToModify"=w742, "VIToAdd"=w744, "error in (no error)"=w743, "AddVIOnLeftSideCaseStructure"=TRUE, "OnlyReference"=TRUE) -> ("error out"=w741:errorcluster)  [unwired: 14 in]
                      }
                      frame True {
                        n331 = call <resource>:"Scripting_AddVIBetweenVIs.vi"("ViToModify"=w748, "VIToAdd"=w751, "VIOne(Path,Name or NamePattern)"="GetInstance.vi" ("regular expression"), "VITwo(Path,Name or NamePattern), If Left/Right-string, it will be placed to the right or left of VIOne"="GetAttributes.vi" ("regular expression"), "error in (no error)"=w750) -> ("error out"=w749:errorcluster)  [unwired: 13 in, 1 out]
                      }
                    }
                    n332 = invoke class="VI" method="Save.Instrument"(reference=w735, error in=w734) -> (reference out=w732:refnum<vi>, error out=w733:errorcluster)  [unwired: 4 in, 4 out]
                    n333 = Close Reference(reference=w732, error in (no error)=w733) -> (error out=w731:errorcluster)
                    n334 = case shown="Error" w731 {
                      selector: w731 -> [w752 _]
                      tunnel: [w752 w754] -> w730
                      tunnel: w729 -> [_ w754]
                      tunnel: w728 -> [_ w753]
                      frame No Error {
                      }
                      frame Error {
                        n335 = One Button Dialog(message=w753) -> ()  [unwired: 1 in, 1 out]
                      }
                    }
                  }
                }
              }
            }
          }
          frame "SaveAll" {
            n336 = call <resource>:"GDSLvClass_SaveEverythingInClass.vi"("ClassRefIn"=w763, "ForceResaving(False)"=TRUE, "error in"=w765) -> ("error out"=w764:errorcluster)  [unwired: 15 in, 1 out]
          }
        }
        n337 = Equal?(x=w160, y="Exit") -> (x = y?=w163:bool)
        n338 = Select(t="Error", s=w159, f=w160) -> (s? t:f=w164:string)
      }
    }
    frame "RemovePattern" {
    }
    frame "UpdatePattern" {
    }
    frame "CreatePatternMethod" {
      w776 = "Init"
      n339 = property class="VI"(error in=w775, "Front Panel.Open"=FALSE ("Front Panel Window:Open")) -> (error out=w777:errorcluster)  [unwired: 1 in, 1 out]
      n340 = while {
        shift-right: [w786] -> w770
        shift-left: w777 -> [w793]
        shift-right: [w791] -> _
        shift-left: w776 -> [w792]
        shift-right: [w779] -> _
        shift-left: _ -> [w785]
        tunnel: w773 -> [w784]
        tunnel: w771 -> [w783]
        tunnel: w772 -> [w782]
        tunnel: w774 -> [w781]
        shift-left: w776 -> [w780]
        stop <- w790 stop-if-true
        n341 = case shown="\"Place_GetInstanceVI\"" w792 {
          tunnel: w793 -> [w822 w840 w862]
          tunnel: [w814 w839 w863] -> w786
          tunnel: [w812 "ReplaceProcessRepositoryVI" "Exit"] -> w787
          tunnel: w785 -> [_ w826 w865]
          tunnel: w784 -> [w823 _ _]
          tunnel: w783 -> [_ _ _]
          tunnel: w782 -> [w803 _ _]
          tunnel: w781 -> [w815 w841 w864]
          tunnel: w780 -> [_ _ _]
          tunnel: [w797 w826 w865] -> w779
          frame "Init" {
            n342 = Variant To Data(error in=w822, type=cluster{path, "VI":refnum<vi>, "Name":string} {path "", "VI"=refnum, "Name"=""} ("cluster"), Variant=w823) -> (data=w805:cluster{path, "VI":refnum<vi>, "Name":string}, error out=w807:errorcluster)
            n343 = Unbundle(w805) -> (w802:path, "VI"=w801:refnum<vi>, "Name"=w794:string)
            n344 = call <resource>:"GDSLvClass_ReadClassType.vi"("Class Refnum In"=w815, "error in (no error)"=w807) -> ("ClassSettings"=w821:T14, "error out"=w814:errorcluster)  [unwired: 15 in, 1 out]
            n345 = Unbundle By Name(w821) -> ("ConnectorPanePattern"=w820:string, "ClassTemplateUsed"=w819:string)
            n346 = To Lower Case(string=w819) -> (all lower case string=w817:string)
            n347 = case shown="\"0\", Default" w820 {
              tunnel: ["4x4x4" "6x8x6"] -> _
              frame "0", Default {
              }
              frame "1", "2" {
              }
            }
            n348 = Match Pattern(string=w817, regular expression="singleton" ("search string")) -> (offset past match=w818:i32)  [unwired: 1 in, 3 out]
            n349 = Greater Or Equal To 0?(x=w818) -> (x >= 0?=w813:bool)
            n350 = Current VI's Path() -> (path=w810:path)
            n351 = Strip Path(path=w810) -> (stripped path=w809:path)  [unwired: 1 out]
            n352 = Build Path(base path=w809, name or relative path="ActiveObjects_DynamicEvents_SubVIs") -> (appended path=w800:path)
            n353 = Build Path(base path=w800, name or relative path="ActiveObjects_DynamicEvents_ProcessRepository_Native.vi") -> (appended path=w798:path)
            n354 = Build Path(base path=w800, name or relative path="ActiveObjects_DynamicEvents_Process.vi") -> (appended path=w795:path)
            n355 = Bundle By Name(cluster=w803, "MethodTemplate"=w802, "VI"=w801, "SupportFolder"=w800, "VI_ToFind"=w798, "VI_ToFindSingleton"=w795, "Name"=w794) -> (w797:T4)
            n356 = Select(t="Place_GetInstanceVI", s=w813, f="ReplaceProcessRepositoryVI") -> (s? t:f=w812:string)
          }
          frame "Place_GetInstanceVI" {
            n357 = Unbundle By Name(w826) -> ("VI_ToFindSingleton"=w831:path, "VI"=w827:refnum<vi>)
            n358 = Build Array(w831) -> (w830:path[])
            n359 = call <resource>:"GDSLvClass_GetClassMethod.vi"("Class Refnum In"=w841, "VINames"=string[] ["GetInstance.vi$"] ("VIsToSerachFor/ViName"), "error in (no error)"=w840) -> ("ViPaths"=w837:path[], "error out"=w832:errorcluster)  [unwired: 13 in, 2 out]
            n360 = call <resource>:"Scripting_FindVisOnDiagram.vi"("ViRef"=w827, "VIsToSerachFor/ViName"=w830, "error in (no error)"=w832) -> ("VisFound"=w834:refnum<vi>[], "error out"=w833:errorcluster)  [unwired: 15 in]
            n361 = Index Array(array=w837) -> (element=w829:path)  [unwired: 1 in]
            n362 = Index Array(array=w834) -> (element=w835:refnum<vi>)  [unwired: 1 in]
            n363 = invoke class="GObj" method="Replace"(reference=w835, error in=w833, "Path"=w829) -> (error out=w828:errorcluster, "Replace"=w836:refnum<vi>)  [unwired: 3 in, 4 out]
            n364 = Close Reference(reference=w834, error in (no error)=w828) -> ()  [unwired: 1 out]
            n365 = Close Reference(reference=w836, error in (no error)=w828) -> (error out=w839:errorcluster)
          }
          frame "ReplaceGetClassAttributes", Default {
            w849 = "Repository.vi$"
            n366 = Unbundle By Name(w865) -> ("VI_ToFind"=w855:path, "VI"=w851:refnum<vi>, "Name"=w850:string)
            n367 = Build Array(w855) -> (w854:path[])
            n368 = Concatenate Strings(w850, w849) -> (w848:string)
            n369 = Build Array(w848, w849) -> (w843:string[])
            n370 = call <resource>:"GDSLvClass_GetClassMethod.vi"("Class Refnum In"=w864, "VINames"=w843, "error in (no error)"=w862) -> ("ViPaths"=w852:path[], "error out"=w853:errorcluster)  [unwired: 13 in, 2 out]
            n371 = Index Array(array=w852) -> (element #1=w845:path, element #2=w846:path)  [unwired: 2 in]
            n372 = Empty String/Path?(string/path=w845) -> (empty?=w847:bool)
            n373 = Select(t=w846, s=w847, f=w845) -> (s? t:f=w844:path)
            n374 = call <resource>:"Scripting_FindVisOnDiagram.vi"("ViRef"=w851, "VIsToSerachFor/ViName"=w854, "error in (no error)"=w853) -> ("VisFound"=w858:refnum<vi>[], "error out"=w857:errorcluster)  [unwired: 15 in]
            n375 = Index Array(array=w858) -> (element=w860:refnum<vi>)  [unwired: 1 in]
            n376 = invoke class="GObj" method="Replace"(reference=w860, error in=w857, "Path"=w844) -> (error out=w861:errorcluster, "Replace"=w859:refnum<vi>)  [unwired: 3 in, 4 out]
            n377 = Close Reference(reference=w858, error in (no error)=w861) -> ()  [unwired: 1 out]
            n378 = Close Reference(reference=w859, error in (no error)=w861) -> (error out=w856:errorcluster)
            n379 = invoke class="VI" method="Save.Instrument"(reference=w851, error in=w856) -> (error out=w863:errorcluster)  [unwired: 4 in, 5 out]
          }
        }
        n380 = Equal?(x=w787, y="Exit") -> (x = y?=w790:bool)
        n381 = Select(t="Error", s=w786, f=w787) -> (s? t:f=w791:string)
      }
    }
  }
  "error out" <- w8
  "DataOut" <- w5
  "Cancelled" <- w6
  "Name" <- w1
